vi "RT Driver VI.vi"(6 "Device Clock":string, 9 "Device Inputs FIFO":refnum<k33>, 10 "Device Outputs FIFO":refnum<k33>, 11 "Device Reference":T1 format="%.0x") -> ()   [LabVIEW 2017, in "SLSC Switch Engine.lvlib"]
uses:
  SLSC Switch Engine.lvlib
  <vilib>/NI Veristand/Custom Device API/Custom Device Item Ref.ctl
  <vilib>/NI Veristand/Custom Device API/Custom Device Channel Type.ctl
  Outputs With Indices.ctl
  Shared/FIFO Indices.ctl
  Includes/SLSCSwitchMessaging.lvlibp/SLSC Switch Consumer/SLSC Switch Consumer.lvclass
  C:/github/niveristand-routing-and-faulting-custom-device/Includes/CDMessaging.lvlibp/Consumer/Abstract Consumer/Abstract Consumer.lvclass
  <vilib>/NI Veristand/Custom Device API/Custom Device API.lvlib
  <vilib>/NI Veristand/Custom Device Tools/Custom Device Utility Library/Custom Device Utility Library.lvlib
  Includes/CDMessaging.lvlibp/Consumer/Abstract Consumer/Abstract Consumer.lvclass
  Shared/SLSC Switch Shared.lvlib
  C:/github/niveristand-routing-and-faulting-custom-device/Includes/CDMessaging.lvlibp/Switch/Abstract Switch Consumer/Abstract Switch Consumer.lvclass
panel:
  in  "Status Channel":dbl
  in  "Initialization Status Notifier":refnum<notifier>
  in  "Status Notifier":refnum<notifier>
  # "Custom Device Template\nv1.0"
  # "Use this template as a starting point for creating a custom device code module. The input controls shown here are specially named controls that the system will use to provide the device loop with data. The controls are not required for the device loop to run. For instance, if the device doesn't produce any output data, then you don't need the Device Outputs FIFO control. If you do use these controls, however, they need to have these exact names to be functional."
  # "SLSC Switch Shared.lvlib:Compiled.Settings.ctlThe optional status notifier element is used to notify the RT engine of the last state of the custom device, and to indicate the device has completed execution. If this control is not used, a default No Error value is returned to the system when the device finishes execution.\n\nNote: This error state is not checked until the system shuts down. Use an output status channel to send more immediate status values to the system."
  # "This optional input can be used to send the VeriStand Engine the final status of the custom device initalization process. If this control exists on the custom device front panel, the VeriStand Engine will wait for a status update before starting up. If the custom device reports an error, that will abort the execution of the current configuration in the VeriStand Engine.\n\nThis control can be deleted if the custom device does not need to send the initialization status update."
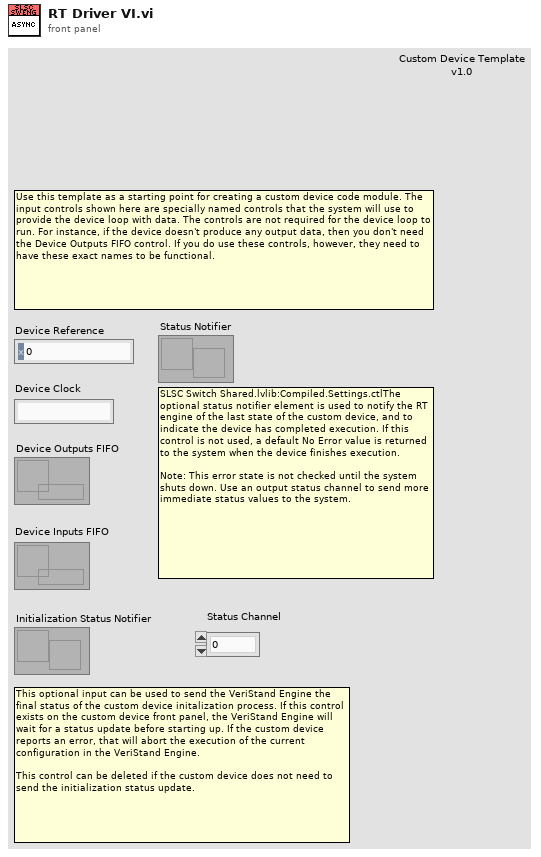
[diagram p1: front panel]
types:
  T1 = typedef "Custom Device API.lvlib/Custom Device Item Ref.ctl" = u64
  T2 = typedef "Custom Device API.lvlib/Custom Device Channel Type.ctl" = enum16{"Input", "Output"}
  T3 = typedef "SLSC Switch Shared.lvlib/FIFO Indices.ctl" = cluster{"Status Channel":i32, "Heartbeat Channel":i32}
  T4 = typedef "Custom Device API.lvlib/Custom Device Engine Event Ref.ctl" = refnum<event-registration>
  T5 = typedef "SLSC Switch Engine.lvlib/Outputs With Indices.ctl" = cluster{"Outputs":dbl[], "FIFO Indices":T3}
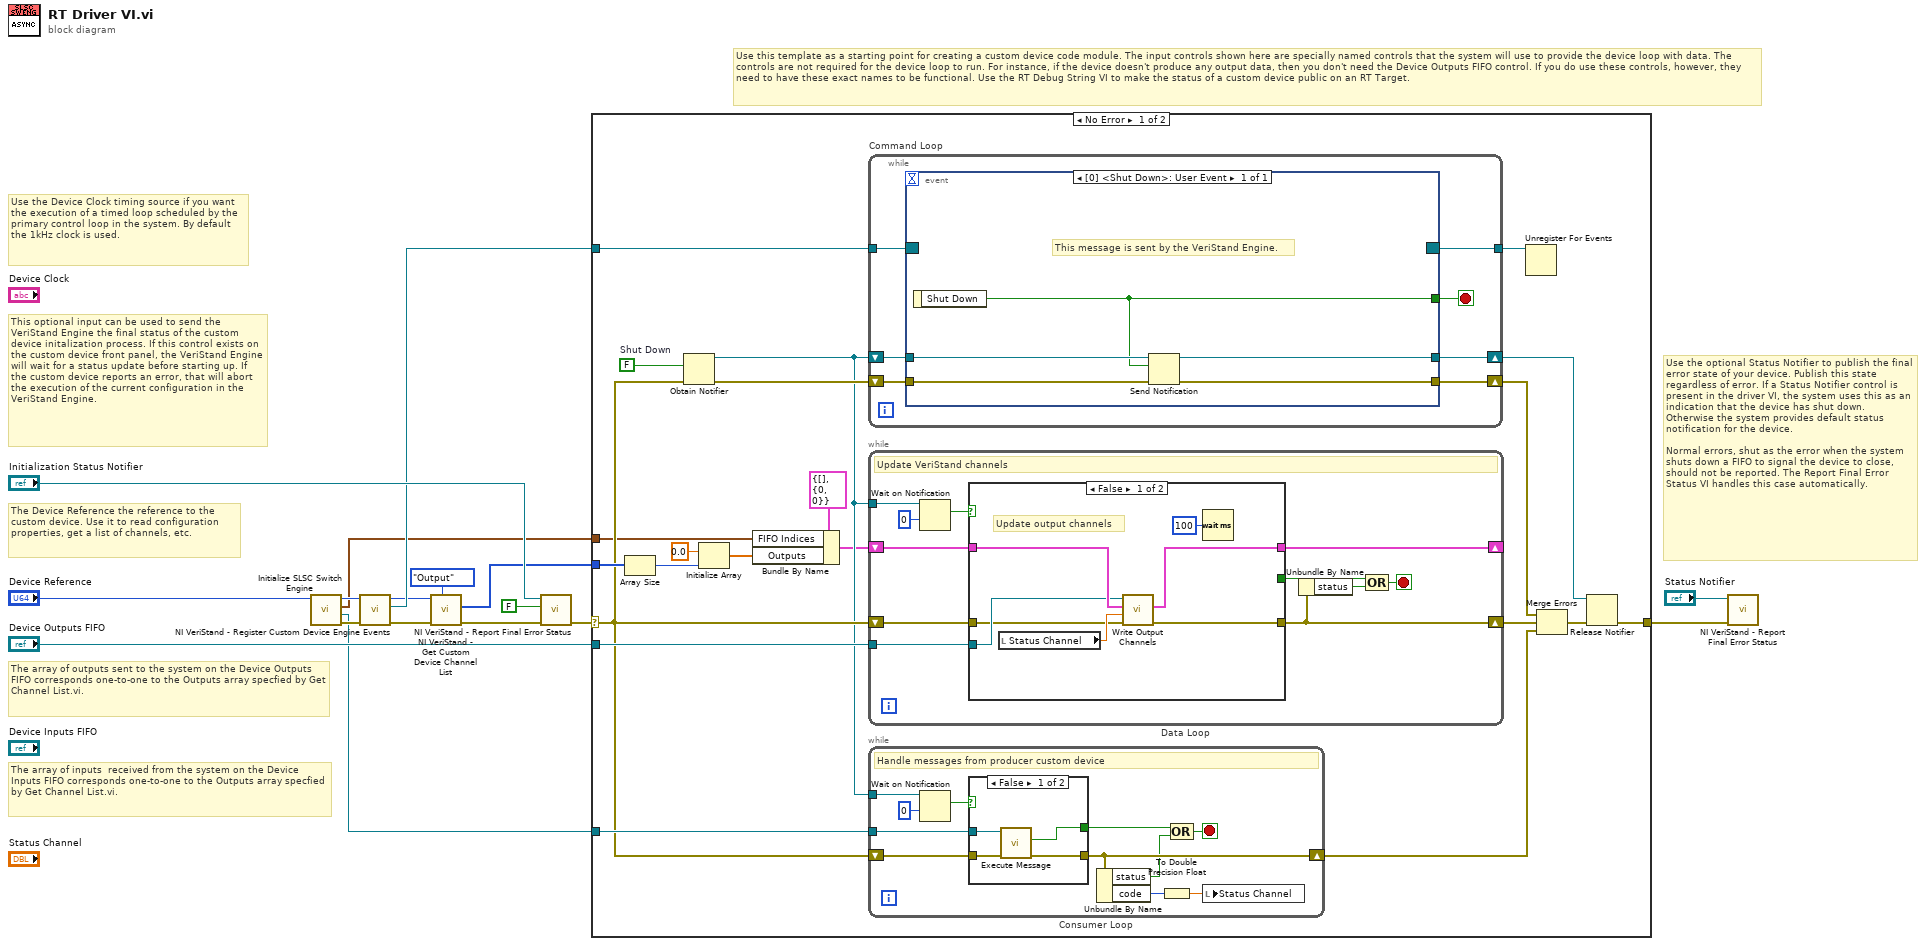
[diagram p0: block diagram]
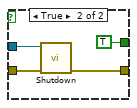
[diagram p2: hidden frame]
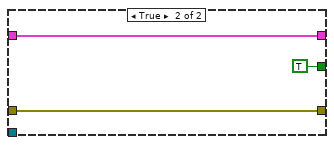
[diagram p3: hidden frame]
diagram:
  # "This optional input can be used to send the VeriStand Engine the final status of the custom device initalization process. If this control exists on the custom device front panel, the VeriStand Engine will wait for a status update before starting up. If the custom device reports an error, that will abort the execution of the current configuration in the VeriStand Engine."
  # "The array of inputs  received from the system on the Device Inputs FIFO corresponds one-to-one to the Outputs array specfied by Get Channel List.vi."
  # "Use the optional Status Notifier to publish the final error state of your device. Publish this state regardless of error. If a Status Notifier control is present in the driver VI, the system uses this as an indication that the device has shut down. Otherwise the system provides default status notification for the device.\n\nNormal errors, shut as the error when the system shuts down a FIFO to signal the device to close, should not be reported. The Report Final Error Status VI handles this case automatically."
  # "The array of outputs sent to the system on the Device Outputs FIFO corresponds one-to-one to the Outputs array specfied by Get Channel List.vi."
  # "The Device Reference the reference to the custom device. Use it to read configuration properties, get a list of channels, etc."
  # "Use the Device Clock timing source if you want the execution of a timed loop scheduled by the primary control loop in the system. By default the 1kHz clock is used."
  # "Use this template as a starting point for creating a custom device code module. The input controls shown here are specially named controls that the system will use to provide the device loop with data. The controls are not required for the device loop to run. For instance, if the device doesn't produce any output data, then you don't need the Device Outputs FIFO control. If you do use these controls, however, they need to have these exact names to be functional. Use the RT Debug String VI to make the status of a custom device public on an RT Target."
  n1 = call "Initialize SLSC Switch Engine.vi"("Device Ref in"="Device Reference") -> ("error out"=w3:errorcluster, "SLSC Switch Consumer out"=w2:refnum<class "SLSC Switch Consumer.lvclass">, "FIFO Indices"=w1:T3, "Device Ref out"=w4:T1)  [unwired: 7 in]
  n2 = call <vilib>:"NI VeriStand - Register Custom Device Engine Events.vi"("error in (no error)"=w3, "Device Ref in"=w4) -> ("error out"=w17:errorcluster, "Custom Device Engine Event Ref"=w10:T4, "Device Ref out"=w8:T1)  [unwired: 7 in]
  n3 = call <vilib>:"NI VeriStand - Get Custom Device Channel List.vi"("Channel Type"=Custom_Device_Channel_Type."Output", "error in (no error)"=w17, "Device Ref in"=w8) -> ("error out"=w13:errorcluster, "Specified Channel Ref List"=w12:T1[])  [unwired: 7 out]
  n4 = call <vilib>:"NI VeriStand - Report Final Error Status.vi"("error in (no error)"=w13, "Filter FIFO & Shutdown Errors (T)"=FALSE ("Filter FIFO Errors (T)"), "Status Notifier"="Initialization Status Notifier") -> ("error out"=w7:errorcluster)  [unwired: 8 out]
  n5 = case shown="No Error" w7 {
    selector: w7 -> [w24 w91]
    tunnel: "Device Outputs FIFO" -> [w37 _]
    tunnel: w12 -> [w34 _]
    tunnel: w10 -> [w33 _]
    tunnel: [w31 w91] -> w9
    tunnel: w2 -> [w25 _]
    tunnel: w1 -> [w20 _]
    frame No Error {
      w32 = FALSE  # Shut Down
      n6 = Array Size(array=w34) -> (size(s)=w35:i32)
      n7 = Obtain Notifier(notification data type=w32, error in (no error)=w24) -> (notifier out=w23:refnum<notifier>, error out=w38:errorcluster)  [unwired: 2 in, 1 out]
      n8 = Initialize Array(0.0 ("element"), w35) -> (w19:dbl[])
      n9 = Bundle By Name(cluster=T5 {"Outputs"=[], "FIFO Indices"={"Status Channel"=0, "Heartbeat Channel"=0}} ("Outputs"), "FIFO Indices"=w20, "Outputs"=w19) -> (w18:T5)
      n10 = while "Command Loop" {
        tunnel: w33 -> [w64]
        tunnel: [w63] -> w30
        shift-right: [w60] -> w29
        shift-left: w23 -> [w61]
        shift-right: [w58] -> w26
        shift-left: w38 -> [w59]
        stop <- w62 stop-if-true
        n11 = event shown="[0] <Shut Down>: User Event" {
          selector: w64 -> [_]
          dyn-events: [_] -> w63
          timeout: _ -> [_]
          tunnel: [w67] -> w62
          tunnel: w61 -> [w68]
          tunnel: [w69] -> w60
          tunnel: w59 -> [w66]
          tunnel: [w65] -> w58
          event User Event {
            # "This message is sent by the VeriStand Engine."
            n12 = event-data() -> ("Shut Down"=w67:bool)  [unwired: 1 in]
            n13 = Send Notification(notification=w67, notifier=w68, error in (no error)=w66) -> (notifier out=w69:refnum<notifier>, error out=w65:errorcluster)
          }
        }
      }
      n14 = while "Data Loop" {
        shift-right: [w75] -> w28
        shift-left: w24 -> [w80]
        shift-right: [w78] -> _
        shift-left: w18 -> [w79]
        tunnel: w37 -> [w77]
        tunnel: w23 -> [w74]
        stop <- w70 stop-if-true
        # "Update VeriStand channels"
        n15 = Wait on Notification(notifier=w74, timeout in ms (-1)=0) -> (notification=w73:bool)  [unwired: 2 in, 3 out]
        n16 = case shown="False" w73 {
          tunnel: w80 -> [w81 w90]
          tunnel: w79 -> [w86 w89]
          tunnel: [w84 w89] -> w78
          tunnel: w77 -> [w83 _]
          tunnel: [w85 w90] -> w75
          tunnel: [_ TRUE] -> w71
          frame False {
            # "Update output channels"
            n17 = local read "Status Channel"() -> (w82:dbl)
            n18 = call "Write Output Channels.vi"("error in (no error)"=w81, "Status"=w82, "Outputs"=w86, "Device Outputs FIFO"=w83) -> ("error out"=w85:errorcluster, "Updated Outputs"=w84:T5)  [unwired: 6 in]
            n19 = Wait (ms)(milliseconds to wait=u32 100) -> ()  [unwired: 1 out]
          }
          frame True {
          }
        }
        n20 = Unbundle By Name(w75) -> ("status"=w72:bool)
        n21 = Compound Arithmetic op=OR(w71, w72) -> (w70:bool)
      }
      n22 = while "Consumer Loop" {
        tunnel: w25 -> [w48]
        shift-right: [w45] -> w22
        shift-left: w24 -> [w46]
        tunnel: w23 -> [w43]
        stop <- w49 stop-if-true
        # "Handle messages from producer custom device"
        n23 = Wait on Notification(notifier=w43, timeout in ms (-1)=0) -> (notification=w42:bool)  [unwired: 2 in, 3 out]
        n24 = case shown="False" w42 {
          tunnel: w48 -> [w53 w56]
          tunnel: [w52 TRUE ("Stop?")] -> w47
          tunnel: w46 -> [w51 w57]
          tunnel: [w50 w55] -> w45
          frame False {
            n25 = call "Execute Message.vi"("error in (no error)"=w51, "Abstract Consumer in"=w53) -> ("error out"=w50:errorcluster, "Stop?"=w52:bool)  [unwired: 7 in, 1 out]
          }
          frame True {
            n26 = call "Shutdown.vi"("error in (no error)"=w57, "Abstract Consumer in"=w56) -> ("error out"=w55:errorcluster)  [unwired: 8 in, 1 out]
          }
        }
        n27 = Unbundle By Name(w45) -> ("status"=w41:bool, "code"=w40:i32)
        n28 = To Double Precision Float(number=w40) -> (double precision float=w39:dbl)
        n29 = Compound Arithmetic op=OR(w47, w41) -> (w49:bool)
        n30 = local write "Status Channel"(w39) -> ()
      }
      n31 = Unregister For Events(event registration refnum=w30) -> ()  [unwired: 1 in, 1 out]
      n32 = Merge Errors(w26, w28, w22) -> (w27:errorcluster)
      n33 = Release Notifier(notifier=w29, error in (no error)=w27) -> (error out=w31:errorcluster)  [unwired: 1 in, 2 out]
    }
    frame Error {
    }
  }
  n34 = call <vilib>:"NI VeriStand - Report Final Error Status.vi"("error in (no error)"=w9, "Status Notifier"="Status Notifier") -> ()  [unwired: 1 in, 9 out]
